vi "Set Single Column Param.vi"(8 "error in (no error)":errorcluster, 9 "Params":string, 10 "column index":i32, 11 "DataTable in":refnum<class "DataTable.lvclass">) -> (0 "error out":errorcluster, 3 "DataTable out":refnum<class "DataTable.lvclass">)   [LabVIEW 2016, in "DataGrid.lvlib" / "DataTable.lvclass"]
uses:
  <userlib>/LabVIEWdotNetDataGrid/source/DataTable/DataTable.lvclass
  <userlib>/LabVIEWdotNetDataGrid/source/DataTable/DataTable.lvclass/DataTable.ctl
  <userlib>/LabVIEWdotNetDataGrid/source/GridColumn/GridColumn.lvclass/GridColumn.ctl
  <userlib>/LabVIEWdotNetDataGrid/source/GridColumn/Write Params.vi
  <userlib>/LabVIEWdotNetDataGrid/source/GridColumn/GridColumn.lvclass
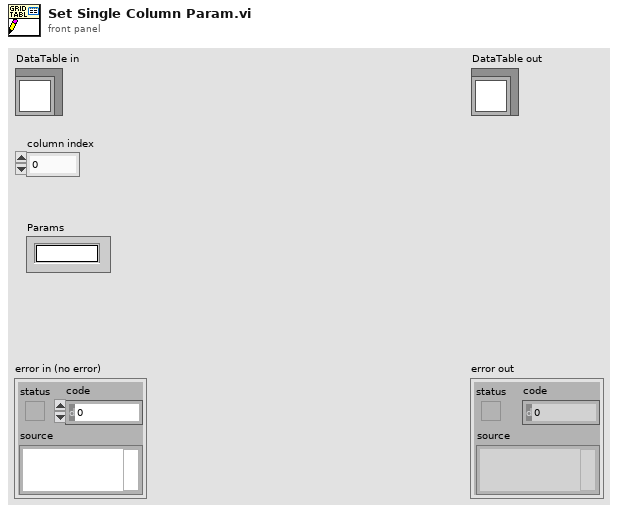
[diagram p1: front panel]
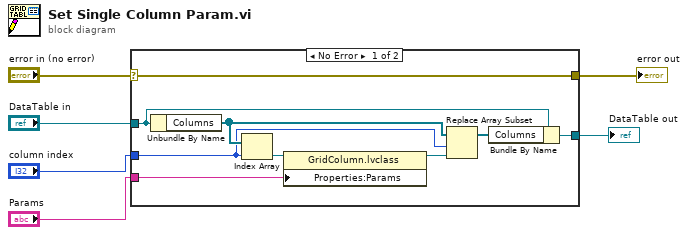
[diagram p0: block diagram]
diagram:
  n1 = case shown="No Error" "error in (no error)" {
    selector: "error in (no error)" -> [w15 w16]
    tunnel: [w15 w16] -> w5
    tunnel: [w14 w17] -> w3
    tunnel: "DataTable in" -> [w13 w17]
    tunnel: "Params" -> [w11 _]
    tunnel: "column index" -> [w9 _]
    frame No Error {
      n2 = Unbundle By Name(w13) -> ("Columns"=w10:refnum<class "GridColumn.lvclass">[])
      n3 = Index Array(array=w10, index=w9) -> (element=w12:refnum<class "GridColumn.lvclass">)
      n4 = property class="GridColumn.lvclass"(reference=w12, "Properties:Params"=w11) -> (reference out=w8:refnum<class "GridColumn.lvclass">)  [unwired: 1 in, 1 out]
      n5 = Replace Array Subset(array=w10, new element=w8, index=w9) -> (w7:refnum<class "GridColumn.lvclass">[])
      n6 = Bundle By Name(cluster=w13, "Columns"=w7) -> (w14:refnum<class "DataTable.lvclass">)
    }
    frame Error {
    }
  }
  "error out" <- w5
  "DataTable out" <- w3
